vi "Rational Resample (multi-channel, DBL).vi"(5 "anti-aliasing?":bool=TRUE, 6 "FIR filter specifications":T1={"alias rejection (dB)"=120.0, "normalized bandwidth"=0.4536} {"normalized bandwidth" format="%.4f"; "alias rejection (dB)" format="%.2f"}, 7 "reset":bool, 8 "error in (no error)":errorcluster, 9 "resample factor":cluster{"interpolation":i32, "decimation":i32}={"interpolation"=1, "decimation"=1}, 10 "start index":i32, 11 "X":dbl[][](array[numeric])) -> (0 "error out":errorcluster, 2 "t0":dbl, 3 "Y":dbl[][](array[numeric]))   [LabVIEW 2017, in "NI_AALPro.lvlib"]
doc: "Resamples the input signal <B>X</B> by interpolating <B>X</B>, passing the interpolated signal through an FIR filter, and decimating the filtered signal. Wire data to the <B>X</B> input to determine the polymorphic instance to use or manually select the instance."
uses:
  NI_AALPro.lvlib
  lvanlys.dll
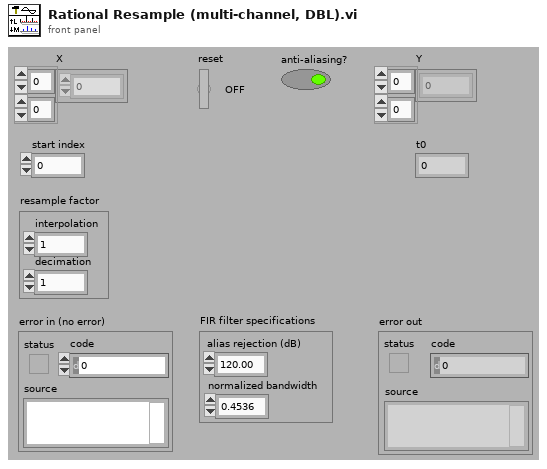
[diagram p1: front panel]
types:
  T1 = cluster{"alias rejection (dB)":dbl, "normalized bandwidth":dbl}
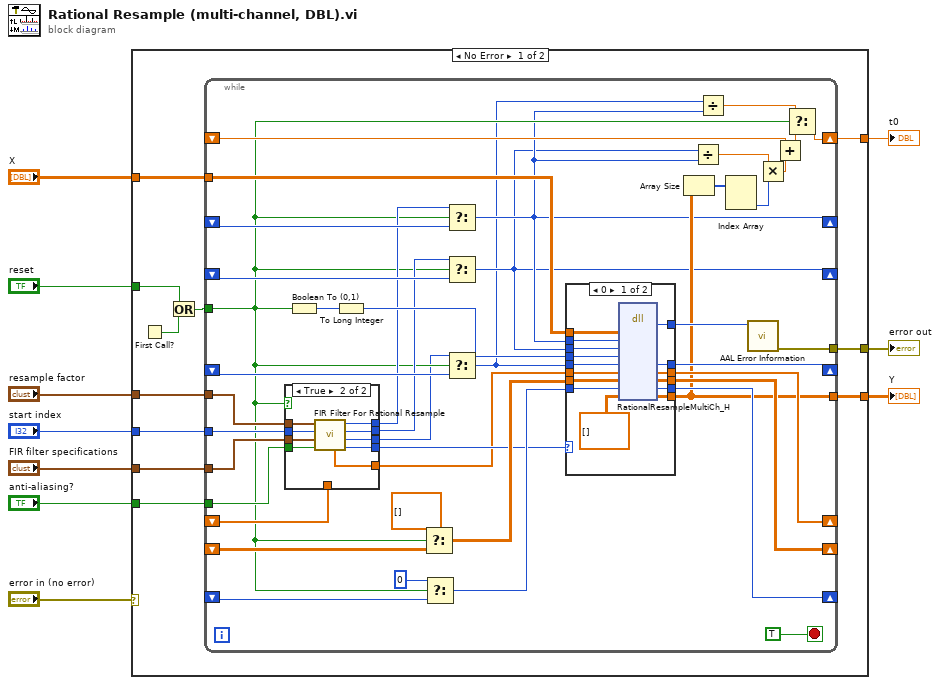
[diagram p0: block diagram]
diagram:
  n1 = case shown="No Error" "error in (no error)" {
    selector: "error in (no error)" -> [_ w90]
    tunnel: "X" -> [w21 _]
    tunnel: "FIR filter specifications" -> [w20 _]
    tunnel: "start index" -> [w19 _]
    tunnel: [w17 w90] -> w8
    tunnel: [w18 _] -> w7
    tunnel: "resample factor" -> [w16 _]
    tunnel: "anti-aliasing?" -> [w15 _]
    tunnel: [w14 _] -> w2
    tunnel: "reset" -> [w11 _]
    frame No Error {
      n2 = First Call?() -> (First Call?: T/F=w13:bool)
      n3 = Or(x=w11, y=w13) -> (x .or. y?=w12:bool)
      n4 = while {
        tunnel: w21 -> [w63]
        shift-right: [w25] -> _
        shift-left: _ -> [w61]
        tunnel: w12 -> [w26]
        shift-right: [w24] -> _
        shift-left: _ -> [w60]
        shift-right: [w44] -> _
        shift-left: _ -> [w57]
        shift-right: [w45] -> _
        shift-left: _ -> [w55]
        shift-right: [w50] -> _
        shift-left: _ -> [w51]
        shift-right: [w48] -> _
        shift-left: _ -> [w47]
        tunnel: w20 -> [w49]
        tunnel: w19 -> [w46]
        tunnel: [w35] -> w18
        tunnel: [w42] -> w17
        tunnel: w16 -> [w41]
        tunnel: w15 -> [w38]
        shift-right: [w36] -> w14
        shift-left: _ -> [w28]
        stop <- TRUE stop-if-true
        n5 = case shown="True" w26 {
          tunnel: [w80 w83] -> w39
          tunnel: w49 -> [_ w84]
          tunnel: w47 -> [w80 _]
          tunnel: [_ w89] -> w31
          tunnel: [_ w88] -> w32
          tunnel: w46 -> [_ w85]
          tunnel: [_ w87] -> w22
          tunnel: w41 -> [_ w86]
          tunnel: [_ w82] -> w40
          tunnel: w38 -> [_ w81]
          frame False {
          }
          frame True {
            n6 = call "FIR Filter For Rational Resample.vi"("anti-aliasing?"=w81, "FIR filter specifications"=w84, "start index"=w85, "resample factor"=w86) -> ("error"=w82:i32, "start index out"=w87:i32, "decimation"=w88:i32, "interpolation out"=w89:i32, "filter coefficients"=w83:dbl[])  [unwired: 3 in]
          }
        }
        n7 = Boolean To (0,1)(Boolean=w26) -> (0, 1=w59:i16)
        n8 = To Long Integer(number=w59) -> (32bit integer=w58:i32)
        n9 = Select(t=dbl[][] [] ("yH"), s=w26, f=w57) -> (s? t:f=w53:dbl[][])
        n10 = Select(t=0, s=w26, f=w55) -> (s? t:f=w54:i32)
        n11 = Select(t=w31, s=w26, f=w61) -> (s? t:f=w25:i32)
        n12 = Select(t=w32, s=w26, f=w60) -> (s? t:f=w24:i32)
        n13 = Select(t=w22, s=w26, f=w51) -> (s? t:f=w23:i32)
        n14 = case shown="0" w40 {
          selector: w40 -> [_ w79]
          tunnel: w63 -> [w78 _]
          tunnel: w25 -> [w77 _]
          tunnel: w24 -> [w76 _]
          tunnel: w58 -> [w75 _]
          tunnel: w54 -> [w73 _]
          tunnel: w53 -> [w72 _]
          tunnel: w23 -> [w71 _]
          tunnel: [w70 _] -> w50
          tunnel: w39 -> [w69 _]
          tunnel: [w68 _] -> w48
          tunnel: [w67 _] -> w45
          tunnel: [w66 _] -> w44
          tunnel: [w65 _] -> w35
          tunnel: [w64 w79] -> w43
          frame 0 {
            n15 = dll-call lib="C:/Program Files/National Instruments/LabVIEW 2017/resource/lvanlys.*" fn="RationalResampleMultiCh_H"("X"=w78, "interpolation"=w77, "decimation"=w76, "reset"=w75, "startIndex"=w71, "filterH"=w69, "bufferH"=w72, "singalSizeInBuffer"=w73, "Y"=dbl[][] [] ("yH")) -> (w64:i32, "startIndex"=w70:i32, "filterH"=w68:dbl[], "bufferH"=w66:dbl[][], "singalSizeInBuffer"=w67:i32, "Y"=w65:dbl[][])  [unwired: 7 in, 2 out]
          }
          frame 1, Default {
          }
        }
        n16 = Array Size(array=w35) -> (size(s)=w34:i32[])
        n17 = Divide(x=w24, y=w25) -> (x/y=w30:dbl)
        n18 = Divide(x=w23, y=w25) -> (x/y=w37:dbl)
        n19 = Index Array(array=w34) -> (element #2=w33:i32)  [unwired: 2 in, 1 out]
        n20 = call "AAL Error Information.vi"("error code"=w43) -> ("error out"=w42:errorcluster)  [unwired: 10 in]
        n21 = Multiply(x=w30, y=w33) -> (x*y=w29:dbl)
        n22 = Add(x=w28, y=w29) -> (x+y=w27:dbl)
        n23 = Select(t=w37, s=w26, f=w27) -> (s? t:f=w36:dbl)
      }
    }
    frame Error {
    }
  }
  "error out" <- w8
  "Y" <- w7
  "t0" <- w2
